vi "Torque_1.vi"() -> ()   [LabVIEW 2020]
uses:
  Support/Controls/Cmd_Mouse Popup.ctl
  Support/Controls/Clst_Initialize Input.ctl
  Support/Controls/Cmd_Var Data IO.ctl
  Variables/Global_Cal Info.vi
  Variables/Global_Constant.vi
panel:
  in  "Measured CCW_ADJ":string[][](table) caption="● 조정후 지시값 (반시계방향)"
  in  "Measured CW_ADJ":string[][](table) caption="● 조정후 지시값 (시계방향)"
  out "Condition 2":string[][](table) caption="○ 분동 세트"
  out "표시방식":string
  in  "Measured CCW":string[][](table) caption="● 토크 측정기 지시값 (반시계방향)"
  in  "측정방향":enum16{"양방향", "시계방향", "반시계방향"}(ring)
  in  "Spec 변경":bool
  in  "Random":bool
  out "Spec":string[][](table)
  out "제목":string
  out "에러 출력":errorcluster
  out "Condition":string[][](table) caption="○ 정확도 교정"
  in  "최소눈금":string(combo)
  out "단위":string
  out "최대용량":string
  in  "Measured CW":string[][](table) caption="● 토크 측정기 지시값 (시계방향)"
  out "Load?":bool
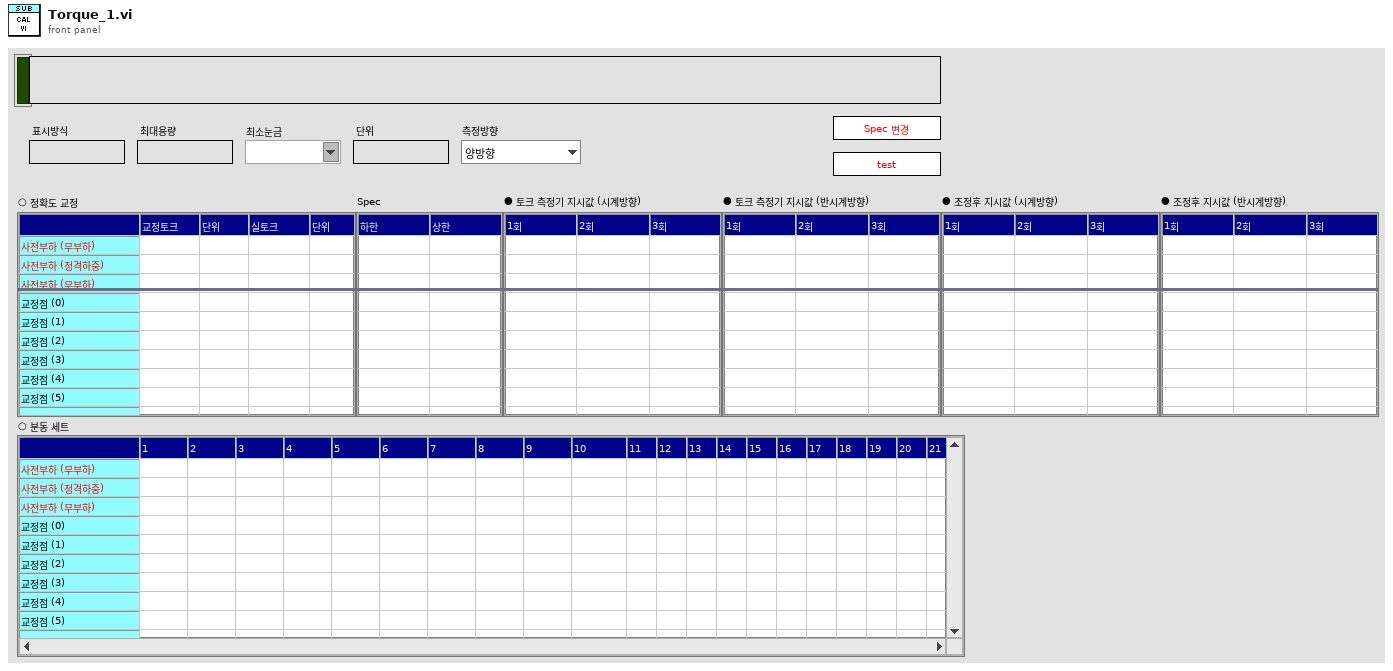
[diagram p1: front panel]
types:
  T1 = typedef "Clst_Cal Info Global.ctl" = cluster{"등록번호":string, "의뢰기관":string, "기기명":string, "제작회사":string, "형식":string, "기기번호":string, "소분류코드":string, "세부분류코드":string, "교정주기":string, "접수번호":string, "교정일자":string, "교정절차서 1":string, "교정절차서 2":string, "교정절차서 3":string, "접수확인자":string, "인증교정자":string, "기술책임자":string, "KOLAS 유무":string, "진행상태":string, "의뢰기관코드":string, "입고형태":string, "영문성적서?":bool, "합불판정?":bool, "부록?":bool, "절차서번호 1":string, "절차서번호 2":string, "절차서번호 3":string, "교정방식":string, "부서명":string}
  T2 = typedef "Cmd_Mouse Popup.ctl" = enum16{"활성화", "메뉴선택"}
  T3 = cluster{"Shift":bool, "Ctrl":bool, "Alt":bool, "Cmd":bool, "Opt":bool}
  T4 = typedef "Clst_Initialize Input.ctl" = cluster{"Initialize 1":cluster{"Condition":refnum<vi>[], "Spec":refnum<vi>[], "Measured":refnum<vi>[], "Resolution":refnum<vi>[], "Func_ext":string, "제목":refnum<vi>, "Measured_ADJ":refnum<vi>[]}, "Initialize 2":cluster{"문자열":refnum<vi>[], "콤보박스":refnum<vi>[], "링":refnum<vi>[], "열거형":refnum<vi>[], "테이블":refnum<vi>[], "여러열":refnum<vi>[], "디지털(DBL)":refnum<vi>[], "3D string":refnum<vi>[], "ctrl":refnum<vi>[], "boolean":refnum<vi>[]}}
  T5 = typedef "Cmd_Var Data IO.ctl" = enum16{"Condition", "Condition Default", "Condition_Temp", "Resolution", "Resolution Default", "Resolution Old", "Spec", "Spec Default", "Spec Old", "Spec Temp", "Result", "Result2", "Result3", "Result_Temp", "Result_ADJ", "Result_ADJ2", "STD1", "STD2", "STD3", "STD4", "STD5", "STD Temp", "CMC", "CMC Default"}
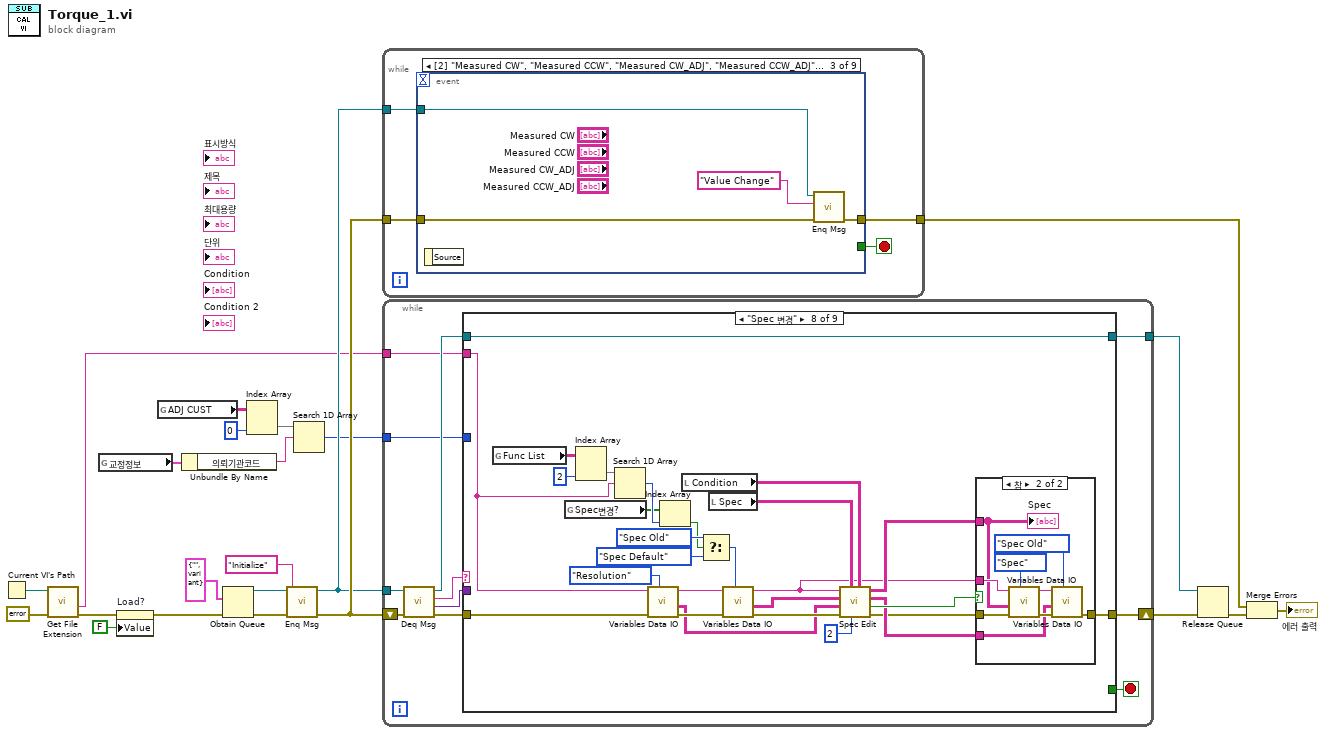
[diagram p0: block diagram]
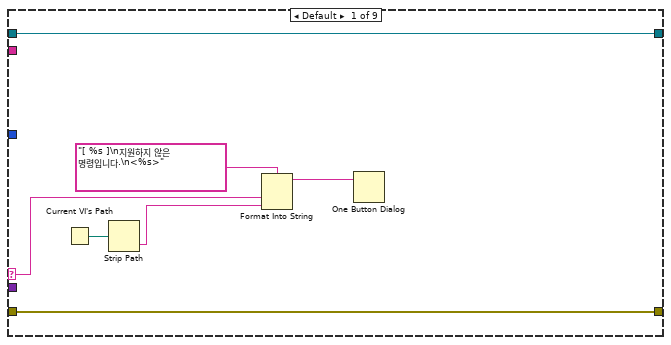
[diagram p2: hidden frame]
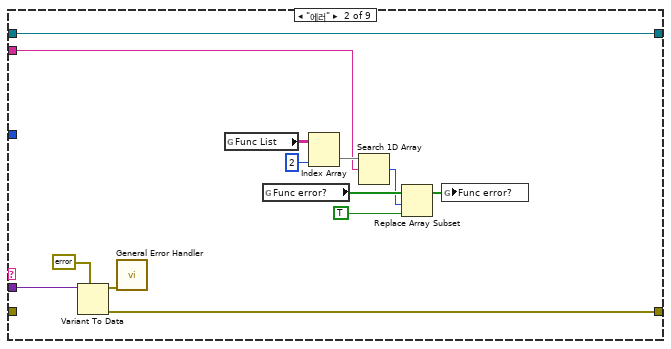
[diagram p3: hidden frame]
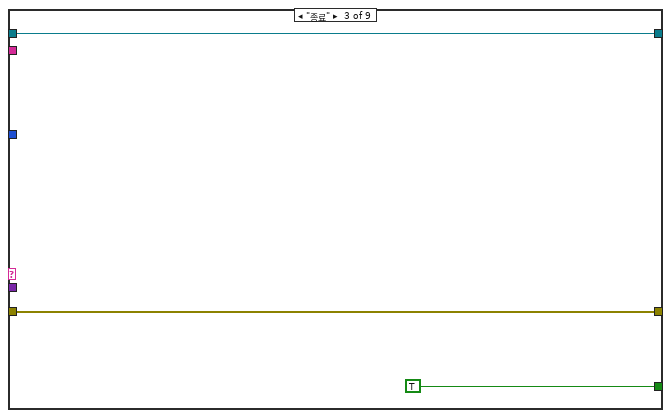
[diagram p4: hidden frame]
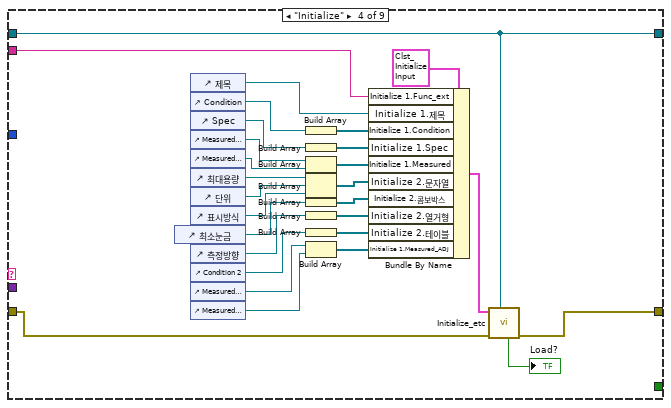
[diagram p5: hidden frame]
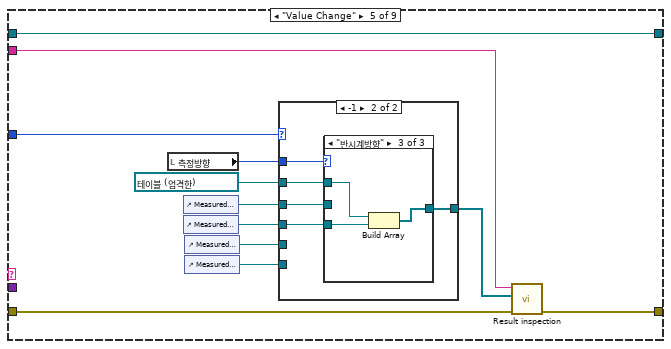
[diagram p6: hidden frame]
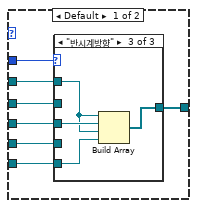
[diagram p7: hidden frame]
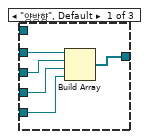
[diagram p8: hidden frame]
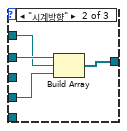
[diagram p9: hidden frame]
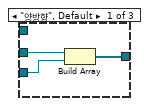
[diagram p10: hidden frame]
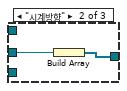
[diagram p11: hidden frame]
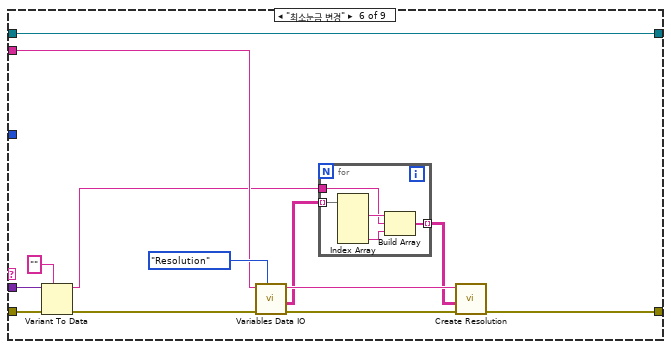
[diagram p12: hidden frame]
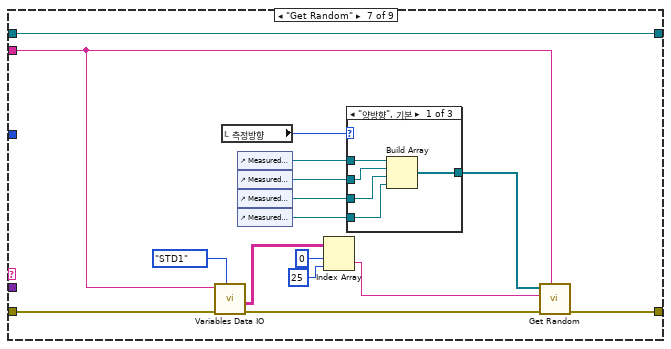
[diagram p13: hidden frame]
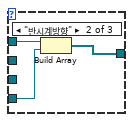
[diagram p14: hidden frame]
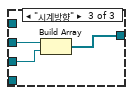
[diagram p15: hidden frame]
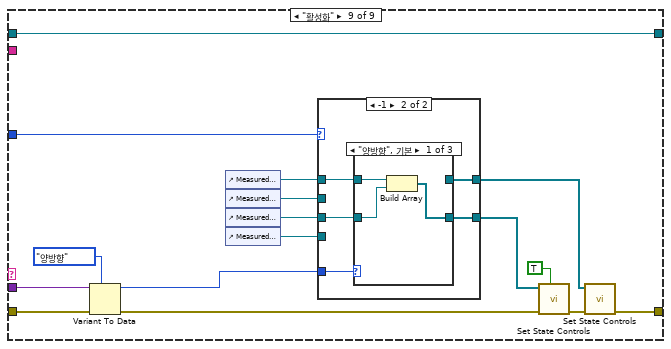
[diagram p17: hidden frame]
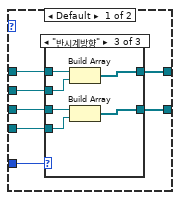
[diagram p18: hidden frame]
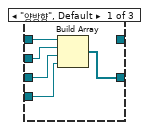
[diagram p19: hidden frame]
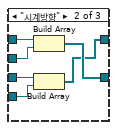
[diagram p20: hidden frame]
diagram:
  n1 = Current VI's Path() -> (path=w11:path)
  n2 = call <vilib>:"Get File Extension.vi"("error in (no error)"=errorcluster {"status"=FALSE, "code"=0, "source"=""} ("에러 상수"), "file"=w11) -> ("error out"=w3:errorcluster, "filename without extension"=w10:string)  [unwired: 5 in, 3 out]
  n3 = global read "Global_Cal Info.vi" "교정정보"() -> (w6:T1)
  n4 = property on="Load?" class="Bool (엄격한)"(error in=w3, "Value"=FALSE ("Load?")) -> (error out=w2:errorcluster)  [unwired: 1 in, 1 out]
  n5 = global read "Global_Constant.vi" "ADJ CUST"() -> (w7:string[][])
  n6 = Unbundle By Name(w6) -> ("의뢰기관코드"=w9:string)
  n7 = Obtain Queue(element data type=cluster{"메세지":string, "값":variant} {"메세지"="", "값"=variant} ("Message Cluster"), error in (no error)=w2) -> (queue out=w20:refnum<queue>, error out=w22:errorcluster)  [unwired: 3 in, 1 out]
  n8 = Index Array(array=w7, index (col)=0 ("비활성화된 인덱스 (열)")) -> (element=w8:string[])  [unwired: 1 in]
  n9 = call "Enq Msg.vi"("에러 입력(에러 없음)"=w22, "메세지"="Initialize", "큐 입력"=w20) -> ("에러 출력"=w21:errorcluster, "큐 출력"=w18:refnum<queue>)  [unwired: 7 in]
  n10 = Search 1D Array(1D array=w8, element=w9) -> (index of element=w4:i32)  [unwired: 1 in]
  n11 = while {
    tunnel: w21 -> [w25]
    tunnel: w18 -> [w26]
    tunnel: [w24] -> w15
    stop <- w27 stop-if-true
    n12 = event shown="[2] \"Measured CW\", \"Measured CCW\", \"Measured CW_ADJ\", \"Measured CCW_ADJ\": 값 변경" {
      selector: _ -> [_ _ _ _ _ _ _ _ _]
      dyn-events: _ -> [_ _ _ _ _ _ _ _ _]
      timeout: _ -> [_ _ _ _ _ _ _ _ _]
      tunnel: [w32 _ _ _ _ _ _ _ _] -> w27
      tunnel: w26 -> [w30 w37 w41 _ w48 _ w62 w68 w78]
      tunnel: w25 -> [w31 w38 w42 w45 w53 w60 w63 w70 w79]
      tunnel: [w28 w35 w39 w44 w47 w59 w61 w69 w73] -> w24
      event Panel Close? {
        w32 = TRUE ("버림?")
        n13 = event-data() -> ()  [unwired: 1 in, 1 out]
        n14 = call "Enq Msg.vi"("에러 입력(에러 없음)"=w31, "메세지"="종료", "큐 입력"=w30) -> ("에러 출력"=w28:errorcluster)  [unwired: 7 in, 1 out]
        n15 = event-data("Discard?"=w32) -> ()  [unwired: 1 in, 1 out]
      }
      event "최소눈금": Value Change {
        n16 = event-data() -> ()  [unwired: 1 in, 1 out]
        n17 = To Variant(anything="최소눈금") -> (Variant=w33:variant)
        n18 = call "Enq Msg.vi"("에러 입력(에러 없음)"=w38, "값"=w33, "메세지"="최소눈금 변경", "큐 입력"=w37) -> ("에러 출력"=w35:errorcluster)  [unwired: 6 in, 1 out]
      }
      event "Measured CW", "Measured CCW", "Measured CW_ADJ", "Measured CCW_ADJ": Value Change {
        n19 = event-data() -> ()  [unwired: 1 in, 1 out]
        n20 = call "Enq Msg.vi"("에러 입력(에러 없음)"=w42, "메세지"="Value Change", "큐 입력"=w41) -> ("에러 출력"=w39:errorcluster)  [unwired: 7 in, 1 out]
      }
      event "Condition", "Spec", "Measured CW", "Measured CCW", "Measured CW_ADJ", "Measured CCW_ADJ": Shortcut Menu Activation? {
        n21 = event-data() -> ("MenuRef"=w43:refnum<k9>)  [unwired: 1 in]
        n22 = call "Mouse PopUp Control.vi"("type"=Cmd_Mouse_Popup."활성화", "error in"=w45, "메뉴 참조"=w43) -> ("error out"=w44:errorcluster)  [unwired: 8 in]
        n23 = event-data() -> ()  [unwired: 2 in, 1 out]
      }
      event "Condition", "Spec", "Measured CW", "Measured CCW", "Measured CW_ADJ", "Measured CCW_ADJ": Shortcut Menu Selection (User) {
        n24 = event-data() -> ("CtlRef"=w51:refnum<vi>, "ItemTag"=w52:string)  [unwired: 1 in]
        n25 = call "Mouse PopUp Control.vi"("type"=Cmd_Mouse_Popup."메뉴선택", "error in"=w53, "아이템 태그"=w52, "Tbl 참조 번호"=w51) -> ("error out"=w49:errorcluster)  [unwired: 7 in]
        n26 = call "Enq Msg.vi"("에러 입력(에러 없음)"=w49, "메세지"="Value Change", "큐 입력"=w48) -> ("에러 출력"=w47:errorcluster)  [unwired: 7 in, 1 out]
      }
      event "Measured CW", "Measured CCW", "Condition", "Measured CW_ADJ", "Measured CCW_ADJ": Key Down; "Measured CW", "Measured CCW", "Condition", "Measured CW_ADJ", "Measured CCW_ADJ": Key Repeat {
        n27 = event-data() -> ("PlatMods"=w55:T3, "ScanCode"=w58:i16, "Mods.Num Pad"=w57:bool, "CtlRef"=w56:refnum<vi>)  [unwired: 1 in]
        n28 = call "Cursor Control.vi"("플랫폼 조합키"=w55, "참조"=w56, "Num Pad"=w57, "ScanCode"=w58, "error in"=w60) -> ("error out"=w59:errorcluster)  [unwired: 5 in, 1 out]
      }
      event "Random": Value Change {
        n29 = event-data() -> ()  [unwired: 1 in, 1 out]
        n30 = call "Enq Msg.vi"("에러 입력(에러 없음)"=w63, "메세지"="Get Random", "큐 입력"=w62) -> ("에러 출력"=w65:errorcluster, "큐 출력"=w66:refnum<queue>)  [unwired: 7 in]
        n31 = call "Enq Msg.vi"("에러 입력(에러 없음)"=w65, "메세지"="Value Change", "큐 입력"=w66) -> ("에러 출력"=w61:errorcluster)  [unwired: 7 in, 1 out]
      }
      event "Spec 변경": Value Change {
        n32 = event-data() -> ()  [unwired: 1 in, 1 out]
        n33 = call "Enq Msg.vi"("에러 입력(에러 없음)"=w70, "메세지"="Spec 변경", "큐 입력"=w68) -> ("에러 출력"=w69:errorcluster)  [unwired: 7 in, 1 out]
      }
      event "측정방향": Value Change {
        n34 = event-data() -> ()  [unwired: 1 in, 1 out]
        n35 = To Variant(anything="측정방향") -> (Variant=w77:variant)
        n36 = call "Enq Msg.vi"("에러 입력(에러 없음)"=w79, "값"=w77, "메세지"="활성화", "큐 입력"=w78) -> ("에러 출력"=w74:errorcluster, "큐 출력"=w72:refnum<queue>)  [unwired: 6 in]
        n37 = call "Enq Msg.vi"("에러 입력(에러 없음)"=w74, "메세지"="Value Change", "큐 입력"=w72) -> ("에러 출력"=w73:errorcluster)  [unwired: 7 in, 1 out]
      }
    }
  }
  n38 = while {
    shift-right: [w91] -> w17
    shift-left: w21 -> [w90]
    tunnel: w18 -> [w88]
    tunnel: [w83] -> w16
    tunnel: w10 -> [w82]
    tunnel: w4 -> [w81]
    stop <- w84 stop-if-true
    n39 = call "Deq Msg.vi"("에러 입력(에러 없음)"=w90, "큐 입력"=w88) -> ("에러 출력"=w89:errorcluster, "값"=w85:variant, "메세지"=w87:string, "큐 출력"=w86:refnum<queue>)  [unwired: 6 in]
    n40 = case shown="\"Spec 변경\"" w87 {
      selector: w87 -> [w94 _ _ _ _ _ _ _ _]
      tunnel: w89 -> [w98 _ w114 w125 w151 w199 w218 w236 w284]
      tunnel: [w98 w108 w114 w122 w153 w191 w220 w237 w278] -> w91
      tunnel: w86 -> [w97 w107 w112 w130 w154 w200 w221 w259 w285]
      tunnel: w85 -> [_ w109 _ _ _ w198 _ _ w283]
      tunnel: [_ _ TRUE ("버림?") _ _ _ _ _ _] -> w84
      tunnel: [w97 w107 w112 w130 w154 w200 w221 w259 w285] -> w83
      tunnel: w82 -> [_ w99 _ w121 w152 w193 w219 w235 _]
      tunnel: w81 -> [_ _ _ _ w143 _ _ _ w270]
      frame Default {
        n41 = Current VI's Path() -> (path=w93:path)
        n42 = Strip Path(path=w93) -> (name=w92:string)  [unwired: 1 out]
        n43 = Format Into String(format string="[ %s ]\n지원하지 않은 명령입니다.\n<%s>" ("메시지"), w94, w92) -> (resulting string=w95:string)  [unwired: 2 in, 1 out]
        n44 = One Button Dialog(message=w95) -> ()  [unwired: 1 in, 1 out]
      }
      frame "에러" {
        n45 = Variant To Data(type=errorcluster {"status"=FALSE, "code"=0, "source"=""} ("에러 출력"), Variant=w109) -> (data=w111:errorcluster, error out=w108:errorcluster)  [unwired: 1 in]
        n46 = call <vilib>:"General Error Handler.vi"("error in (no error)"=w111) -> ()  [unwired: 10 in, 5 out]
        n47 = global read "Global_Cal Info.vi" "Func List"() -> (w105:string[][])
        n48 = global read "Global_Cal Info.vi" "Func error?"() -> (w102:bool[])
        n49 = Index Array(array=w105, index (col)=2 ("비활성화된 인덱스 (열)")) -> (element=w104:string[])  [unwired: 1 in]
        n50 = Search 1D Array(1D array=w104, element=w99) -> (index of element=w101:i32)  [unwired: 1 in]
        n51 = Replace Array Subset(array=w102, new element=TRUE ("새 원소/부분배열"), index=w101) -> (w100:bool[])
        n52 = global write "Global_Cal Info.vi" "Func error?"(w100) -> ()
      }
      frame "종료" {
      }
      frame "Initialize" {
        n53 = control-ref of="최소눈금"() -> (w136:refnum<vi>)
        n54 = control-ref of="제목"() -> (w134:refnum<vi>)
        n55 = control-ref of="Condition"() -> (w129:refnum<vi>)
        n56 = control-ref of="Spec"() -> (w124:refnum<vi>)
        n57 = control-ref of="Measured CW"() -> (w138:refnum<vi>)
        n58 = control-ref of="Measured CCW"() -> (w128:refnum<vi>)
        n59 = control-ref of="최대용량"() -> (w133:refnum<vi>)
        n60 = control-ref of="단위"() -> (w132:refnum<vi>)
        n61 = control-ref of="표시방식"() -> (w123:refnum<vi>)
        n62 = control-ref of="측정방향"() -> (w126:refnum<vi>)
        n63 = control-ref of="Condition 2"() -> (w119:refnum<vi>)
        n64 = control-ref of="Measured CW_ADJ"() -> (w117:refnum<vi>)
        n65 = control-ref of="Measured CCW_ADJ"() -> (w116:refnum<vi>)
        n66 = Build Array(w129) -> (w140:refnum<vi>[])
        n67 = Build Array(w124) -> (w131:refnum<vi>[])
        n68 = Build Array(w138, w128) -> (w139:refnum<vi>[])
        n69 = Build Array(w133, w132, w123) -> (w137:refnum<vi>[])
        n70 = Build Array(w136) -> (w135:refnum<vi>[])
        n71 = Build Array(w126) -> (w127:refnum<vi>[])
        n72 = Build Array(w119) -> (w120:refnum<vi>[])
        n73 = Build Array(w117, w116) -> (w118:refnum<vi>[])
        n74 = Bundle By Name(cluster=T4 {"Initialize 1"={"Condition"=[], "Spec"=[], "Measured"=[], "Resolution"=[], "Func_ext"="", "제목"=refnum, "Measured_ADJ"=[]}, "Initialize 2"={"문자열"=[], "콤보박스"=[], "링"=[], "열거형"=[], "테이블"=[], "여러열"=[], "디지털(DBL)"=[], "3D string"=[], "ctrl"=[], "boolean"=[]}} ("입력 클러스터"), "Initialize 1.Func_ext"=w121, "Initialize 1.제목"=w134, "Initialize 1.Condition"=w140, "Initialize 1.Spec"=w131, "Initialize 1.Measured"=w139, "Initialize 2.문자열"=w137, "Initialize 2.콤보박스"=w135, "Initialize 2.열거형"=w127, "Initialize 2.테이블"=w120, "Initialize 1.Measured_ADJ"=w118) -> (w141:T4)
        n75 = call "Initialize_etc.vi"("큐 입력"=w130, "error in"=w125, "입력 클러스터"=w141) -> ("error out"=w122:errorcluster, "Load?"=→"Load?":bool)  [unwired: 6 in, 1 out]
      }
      frame "Value Change" {
        n76 = local read "측정방향"() -> (w149:enum16{"양방향", "시계방향", "반시계방향"})
        n77 = control-ref of="Measured CW"() -> (w147:refnum<vi>)
        n78 = control-ref of="Measured CCW"() -> (w146:refnum<vi>)
        n79 = control-ref of="Measured CW_ADJ"() -> (w145:refnum<vi>)
        n80 = control-ref of="Measured CCW_ADJ"() -> (w144:refnum<vi>)
        n81 = case shown="-1" w143 {
          tunnel: [w161 w179] -> w150
          tunnel: w149 -> [w160 w178]
          tunnel: refnum<vi> refnum ("Measured CW") -> [w159 w177]
          tunnel: w147 -> [w158 w176]
          tunnel: w146 -> [w157 w175]
          tunnel: w145 -> [w156 _]
          tunnel: w144 -> [w155 _]
          frame Default {
            n82 = case shown="\"반시계방향\"" w160 {
              tunnel: w158 -> [w166 w170 _]
              tunnel: [w165 w169 w174] -> w161
              tunnel: w157 -> [w164 _ w172]
              tunnel: w159 -> [_ w168 w171]
              tunnel: w156 -> [w163 w167 _]
              tunnel: w155 -> [w162 _ w173]
              frame "양방향", Default {
                n83 = Build Array(w166, w164, w163, w162) -> (w165:refnum<vi>[])
              }
              frame "시계방향" {
                n84 = Build Array(w170, w168, w167) -> (w169:refnum<vi>[])
              }
              frame "반시계방향" {
                n85 = Build Array(w171, w172, w171, w173) -> (w174:refnum<vi>[])
              }
            }
          }
          frame -1 {
            n86 = case shown="\"반시계방향\"" w178 {
              tunnel: w176 -> [w182 w184 _]
              tunnel: [w181 w183 w187] -> w179
              tunnel: w175 -> [w180 _ w186]
              tunnel: w177 -> [_ _ w185]
              frame "양방향", Default {
                n87 = Build Array(w182, w180) -> (w181:refnum<vi>[])
              }
              frame "시계방향" {
                n88 = Build Array(w184) -> (w183:refnum<vi>[])
              }
              frame "반시계방향" {
                n89 = Build Array(w185, w186) -> (w187:refnum<vi>[])
              }
            }
          }
        }
        n90 = call "Result inspection.vi"("error in"=w151, "Ref. Data (Inspection)"=w150, "Func ext"=w152) -> ("error out"=w153:errorcluster)  [unwired: 5 in, 3 out]
      }
      frame "최소눈금 변경" {
        n91 = Variant To Data(error in=w199, type="", Variant=w198) -> (data=w190:string, error out=w192:errorcluster)
        n92 = call "Variables Data IO.vi"("Select"=Cmd_Var_Data_IO."Resolution", "error in"=w192, "Func_ext"=w193) -> ("error out"=w195:errorcluster, "Data Out"=w189:string[][], "Func_ext Out"=w194:string)  [unwired: 6 in]
        n93 = for {
          tunnel: w189 -> [w205] mode=indexing
          tunnel: w190 -> [w203]
          tunnel: [w201] -> w188 mode=indexing
          n94 = Index Array(array=w205) -> (element #1=w204:string, element #4=w202:string)  [unwired: 4 in, 2 out]
          n95 = Build Array(w204, w203, w202) -> (w201:string[])
        }
        n96 = call "Create Resolution.vi"("에러 입력(에러 없음)"=w195, "Resolution"=w188, "Func_ext"=w194) -> ("에러 출력"=w191:errorcluster)  [unwired: 6 in, 2 out]
      }
      frame "Get Random" {
        n97 = call "Variables Data IO.vi"("Select"=Cmd_Var_Data_IO."STD1", "error in"=w218, "Func_ext"=w219) -> ("error out"=w217:errorcluster, "Data Out"=w215:string[][])  [unwired: 6 in, 1 out]
        n98 = local read "측정방향"() -> (w210:enum16{"양방향", "시계방향", "반시계방향"})
        n99 = control-ref of="Measured CCW"() -> (w209:refnum<vi>)
        n100 = control-ref of="Measured CW"() -> (w208:refnum<vi>)
        n101 = control-ref of="Measured CW_ADJ"() -> (w207:refnum<vi>)
        n102 = control-ref of="Measured CCW_ADJ"() -> (w206:refnum<vi>)
        n103 = Index Array(array=w215, index (row)=0 ("인덱스 (행)"), index (col)=25 ("비활성화된 인덱스 (열)")) -> (element=w212:string)
        n104 = case shown="\"양방향\", 기본" w210 {
          tunnel: [w226 w229 w232] -> w211
          tunnel: w209 -> [w225 w228 _]
          tunnel: w208 -> [w224 _ w231]
          tunnel: w207 -> [w223 _ w230]
          tunnel: w206 -> [w222 w227 _]
          frame "양방향", Default {
            n105 = Build Array(w225, w224, w223, w222) -> (w226:refnum<vi>[])
          }
          frame "반시계방향" {
            n106 = Build Array(w228, w227) -> (w229:refnum<vi>[])
          }
          frame "시계방향" {
            n107 = Build Array(w231, w230) -> (w232:refnum<vi>[])
          }
        }
        n108 = call "Get Random.vi"("Func_Ext"=w219, "에러 입력"=w217, "분해능"=w212, "Meas"=w211) -> ("에러 출력"=w220:errorcluster)  [unwired: 6 in, 1 out]
      }
      frame "Spec 변경" {
        n109 = global read "Global_Cal Info.vi" "Func List"() -> (w243:string[][])
        n110 = global read "Global_Cal Info.vi" "Spec변경?"() -> (w239:bool[])
        n111 = Index Array(array=w243, index (col)=2 ("비활성화된 인덱스 (열)")) -> (element=w241:string[])  [unwired: 1 in]
        n112 = Search 1D Array(1D array=w241, element=w235) -> (index of element=w240:i32)  [unwired: 1 in]
        n113 = call "Variables Data IO.vi"("Select"=Cmd_Var_Data_IO."Resolution", "error in"=w236, "Func_ext"=w235) -> ("error out"=w250:errorcluster, "Data Out"=w233:string[][], "Func_ext Out"=w249:string)  [unwired: 6 in]
        n114 = Index Array(array=w239, index=w240) -> (element=w244:bool)
        n115 = local read "Condition"() -> (w253:string[][])
        n116 = Select(t=Cmd_Var_Data_IO."Spec Old" ("Select"), s=w244, f=Cmd_Var_Data_IO."Spec Default" ("Select")) -> (s? t:f=w238:T5)
        n117 = local read "Spec"() -> (w254:string[][])
        n118 = call "Variables Data IO.vi"("Select"=w238, "error in"=w250, "Func_ext"=w249) -> ("error out"=w248:errorcluster, "Data Out"=w234:string[][], "Func_ext Out"=w251:string)  [unwired: 6 in]
        n119 = call "Spec Edit.vi"("Condition"=w253, "열번호(기준값)"=2 ("기준열(0)"), "Spec Value"=w254, "에러 입력(에러 없음)"=w248, "Resolution"=w233, "Spec Default"=w234, "Func_ext"=w251) -> ("에러 출력"=w252:errorcluster, "변경?"=w258:bool, "Spec Default out"=w257:string[][], "Spec 출력"=w255:string[][])  [unwired: 1 in]
        n120 = case shown="참" w258 {
          tunnel: w252 -> [w260 w268]
          tunnel: [w260 w265] -> w237
          tunnel: w255 -> [_ w261]
          tunnel: w251 -> [_ w267]
          tunnel: w257 -> [_ w262]
          frame False {
          }
          frame True {
            n121 = call "Variables Data IO.vi"("Select"=Cmd_Var_Data_IO."Spec", "error in"=w268, "Data In"=w261, "Func_ext"=w267) -> ("error out"=w266:errorcluster, "Func_ext Out"=w263:string)  [unwired: 5 in, 1 out]
            n122 = call "Variables Data IO.vi"("Select"=Cmd_Var_Data_IO."Spec Old", "error in"=w266, "Data In"=w262, "Func_ext"=w263) -> ("error out"=w265:errorcluster)  [unwired: 5 in, 2 out]
            "Spec" <- w261
          }
        }
      }
      frame "활성화" {
        n123 = Variant To Data(error in=w284, type=enum16{"양방향", "시계방향", "반시계방향"}."양방향" ("측정방향 2"), Variant=w283) -> (data=w274:enum16{"양방향", "시계방향", "반시계방향"}, error out=w281:errorcluster)
        n124 = control-ref of="Measured CW"() -> (w275:refnum<vi>)
        n125 = control-ref of="Measured CW_ADJ"() -> (w272:refnum<vi>)
        n126 = control-ref of="Measured CCW"() -> (w273:refnum<vi>)
        n127 = control-ref of="Measured CW_ADJ"() -> (w271:refnum<vi>)
        n128 = case shown="-1" w270 {
          tunnel: [w292 w314] -> w277
          tunnel: [w291 w313] -> w276
          tunnel: w275 -> [w290 w312]
          tunnel: w274 -> [w289 w311]
          tunnel: w273 -> [w288 w310]
          tunnel: w272 -> [w287 _]
          tunnel: w271 -> [w286 _]
          frame Default {
            n129 = case shown="\"반시계방향\"" w289 {
              tunnel: w290 -> [w297 w303 w309]
              tunnel: w288 -> [w296 w301 w308]
              tunnel: [w295 w302 w307] -> w291
              tunnel: [_ w300 w306] -> w292
              tunnel: w287 -> [w294 w299 w305]
              tunnel: w286 -> [w293 w298 w304]
              frame "양방향", Default {
                n130 = Build Array(w297, w294, w296, w293) -> (w295:refnum<vi>[])
              }
              frame "시계방향" {
                n131 = Build Array(w303, w299) -> (w302:refnum<vi>[])
                n132 = Build Array(w301, w298) -> (w300:refnum<vi>[])
              }
              frame "반시계방향" {
                n133 = Build Array(w309, w305) -> (w306:refnum<vi>[])
                n134 = Build Array(w308, w304) -> (w307:refnum<vi>[])
              }
            }
          }
          frame -1 {
            n135 = case shown="\"양방향\", 기본" w311 {
              tunnel: w312 -> [w317 w321 w325]
              tunnel: w310 -> [w316 w319 w324]
              tunnel: [w315 w320 w323] -> w313
              tunnel: [_ w318 w322] -> w314
              frame "양방향", Default {
                n136 = Build Array(w317, w316) -> (w315:refnum<vi>[])
              }
              frame "시계방향" {
                n137 = Build Array(w321) -> (w320:refnum<vi>[])
                n138 = Build Array(w319) -> (w318:refnum<vi>[])
              }
              frame "반시계방향" {
                n139 = Build Array(w325) -> (w322:refnum<vi>[])
                n140 = Build Array(w324) -> (w323:refnum<vi>[])
              }
            }
          }
        }
        n141 = call "Set State Controls.vi"("활성화 (F)"=TRUE, "error in (no error)"=w281, "컨트롤 참조 배열 in"=w276) -> ("error out"=w279:errorcluster)  [unwired: 7 in, 1 out]
        n142 = call "Set State Controls.vi"("error in (no error)"=w279, "컨트롤 참조 배열 in"=w277) -> ("error out"=w278:errorcluster)  [unwired: 8 in, 1 out]
      }
    }
  }
  n143 = Release Queue(queue=w16, error in (no error)=w17) -> (error out=w14:errorcluster)  [unwired: 1 in, 2 out]
  n144 = Merge Errors(w15, w14) -> (→"에러 출력":errorcluster)
